vi "S2C_ExeScriptStatus.vi"(8 "Error In":errorcluster, 11 "Status":T1) -> (0 "Error Out":errorcluster)   [LabVIEW 2015]
doc: "Sets the cell background and font color for the execution table results cell."
uses:
  Controls/S2C_ResultStatus.ctl
  Globals/S2C_Globals.vi
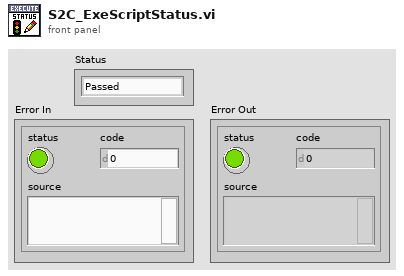
[diagram p1: front panel]
types:
  T1 = typedef "S2C_ResultStatus.ctl" = enum16{"Passed", "Failed", "Logged", "Aborted", "Error", "Testing...", "Paused", "No Record"}
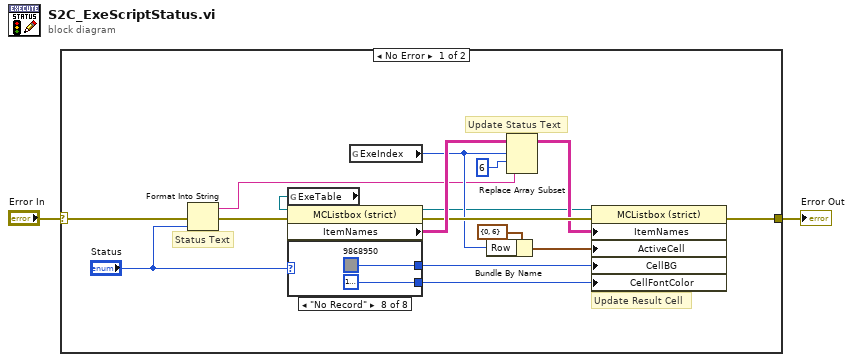
[diagram p0: block diagram]
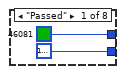
[diagram p2: hidden frame]
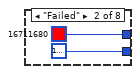
[diagram p3: hidden frame]
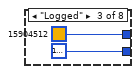
[diagram p4: hidden frame]
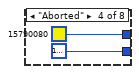
[diagram p5: hidden frame]
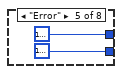
[diagram p6: hidden frame]
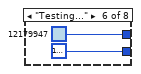
[diagram p7: hidden frame]
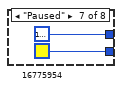
[diagram p8: hidden frame]
diagram:
  n1 = case shown="No Error" "Error In" {
    selector: "Error In" -> [w17 w35]
    tunnel: [w18 w35] -> w1
    frame No Error {
      # "Update Status Text"
      # "Update Result Cell"
      # "Status Text"
      n2 = Format Into String(error in=w17, "Status") -> (resulting string=w5:string, error out=w6:errorcluster)  [unwired: 2 in]
      n3 = global read "S2C_Globals.vi" "ExeTable"() -> (w8:refnum<vi>)
      n4 = property on="Property Node" class="MCListbox (strict)"(reference=w8, error in=w6) -> (reference out=w7:refnum<vi>, error out=w13:errorcluster, "ItemNames"=w15:string[][])
      n5 = case shown="\"No Record\"" "Status" {
        tunnel: [u32 46081 u32 16711680 u32 15904512 u32 15790080 u32 16777222 u32 12179947 u32 16777222 u32 9868950] -> w4
        tunnel: [u32 16777226 u32 16777226 u32 16777226 u32 16777222 u32 16777226 u32 16777222 u32 16775954 u32 16777226] -> w3
        frame "Passed" {
        }
        frame "Failed" {
        }
        frame "Logged" {
        }
        frame "Aborted" {
        }
        frame "Error" {
        }
        frame "Testing..." {
        }
        frame "Paused" {
        }
        frame "No Record" {
        }
      }
      n6 = global read "S2C_Globals.vi" "ExeIndex"() -> (w9:i32)
      n7 = Bundle By Name(cluster=cluster{"Row":i32, "Column":i32} {"Row"=0, "Column"=6} ("Active Cell:Active Cell"), "Row"=w9) -> (w10:cluster{"Row":i32, "Column":i32})
      n8 = Replace Array Subset(array=w15, new element=w5, index (row)=w9, index (col)=6 ("disabled index (col)")) -> (w12:string[][])
      n9 = property on="Property Node" class="MCListbox (strict)"(reference=w7, error in=w13, "ItemNames"=w12, "ActiveCell"=w10, "CellBG"=w4, "CellFontColor"=w3) -> (error out=w18:errorcluster)  [unwired: 1 out]
    }
    frame Error {
    }
  }
  "Error Out" <- w1
